vi "Read Parent.vi"(8 "error in (no error)":errorcluster, 11 "[MDI] Parent in":refnum<class "[MDI] Parent.lvclass">) -> (0 "error out":errorcluster, 2 "parent":refnum<k24>, 3 "[MDI] Parent out":refnum<class "[MDI] Parent.lvclass">)   [LabVIEW 2020, in "[MDI] Parent.lvlib" / "[MDI] Parent.lvclass"]
uses:
  [MDI] Parent.lvclass
  System.Windows.Forms
  [MDI] Parent.lvclass/[MDI] Parent.ctl
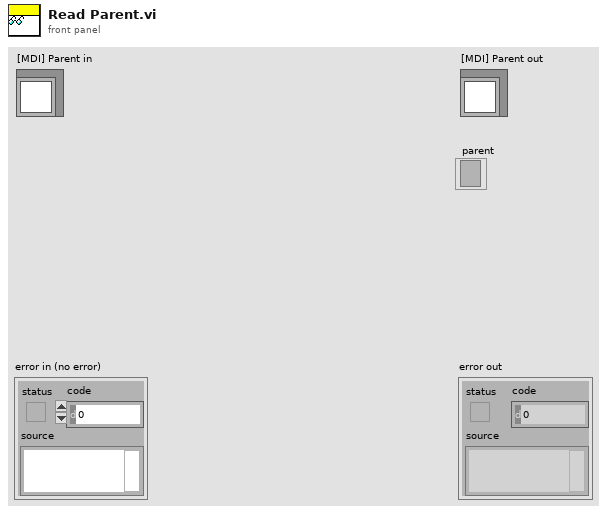
[diagram p1: front panel]
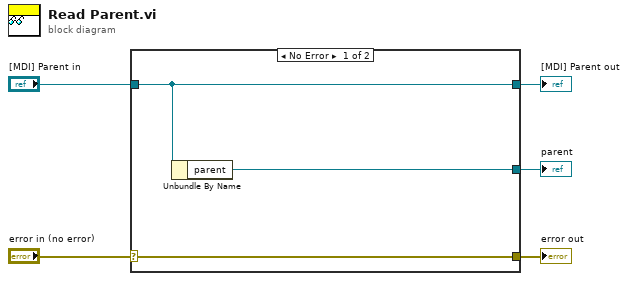
[diagram p0: block diagram]
diagram:
  n1 = case shown="No Error" "error in (no error)" {
    selector: "error in (no error)" -> [w8 w9]
    tunnel: [w8 w9] -> w4
    tunnel: [w7 w10] -> w2
    tunnel: "[MDI] Parent in" -> [w7 w10]
    tunnel: [w6 _] -> w1
    frame No Error {
      n2 = Unbundle By Name(w7) -> ("parent"=w6:refnum<k24>)
    }
    frame Error {
    }
  }
  "error out" <- w4
  "[MDI] Parent out" <- w2
  "parent" <- w1
